vi "Read Magic.vi"(8 "Error In":errorcluster, 11 "Known Host In":refnum<class "Known Host.lvclass">) -> (0 "Error Out":errorcluster, 2 "Magic":i32, 3 "Known Host Out":refnum<class "Known Host.lvclass">)   [LabVIEW 2021, in "Field_RnD_Services_LIBSSH2_Toolkit.lvlib" / "Known Host.lvclass"]
doc: "Gets the \"magic\" number that is part of the libssh2 shared library implementation of a Known Host struct."
uses:
  Known Host.lvclass
  Known Host.lvclass/Known Host.ctl
  Field_RnD_Services_LIBSSH2_Toolkit.lvlib
  SSH/SSH.lvclass
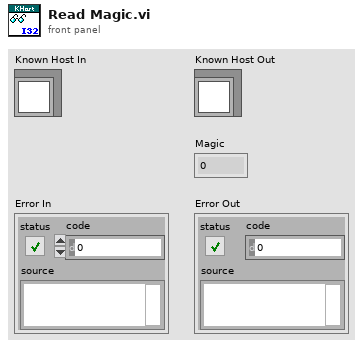
[diagram p1: front panel]
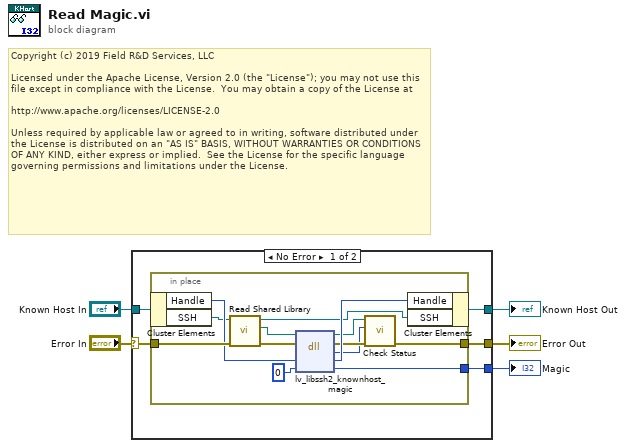
[diagram p0: block diagram]
diagram:
  # "Copyright (c) 2019 Field R&D Services, LLC\n\nLicensed under the Apache License, Version 2.0 (the \"License\"); you may not use this file except in compliance with the License.  You may obtain a copy of the License at\n\nhttp://www.apache.org/licenses/LICENSE-2.0\n\nUnless required by applicable law or agreed to in writing, software distributed under the License is distributed on an \"AS IS\" BASIS, WITHOUT WARRANTIES OR CONDITIONS OF ANY KIND, either express or implied.  See the License for the specific language governing permissions and limitations under the License."
  n1 = case shown="No Error" "Error In" {
    selector: "Error In" -> [w10 w25]
    tunnel: [w9 w25] -> w4
    tunnel: "Known Host In" -> [w8 w24]
    tunnel: [w7 w24] -> w2
    tunnel: [w6 _] -> w1
    frame No Error {
      n2 = in-place {
        in-place-border: w10 -> [w23]
        in-place-border: [w18] -> w9
        in-place-border: [w15] -> w6
        n3 = in-place-cluster #1(w8) -> ("Handle"=w22:u64, "SSH"=w13:refnum<class "SSH.lvclass">)
        n4 = call "Read Shared Library.vi"("Error In"=w23, "SSH In"=w13) -> ("Error Out"=w14:errorcluster, "libssh2lv Shared Library"=w12:path, "SSH Out"=w11:refnum<class "SSH.lvclass">)  [unwired: 7 in]
        n5 = dll-call lib="lv-libssh2.*" fn="lv_libssh2_knownhost_magic"(path in=w12, error in=w14, "handle"=w22, "magic"=0) -> (path out=w17:path, error out=w19:errorcluster, "status"=w16:i32, "handle"=w21:u64, "magic"=w15:i32)  [unwired: 1 in]
        n6 = call "Check Status.vi"("Error In"=w19, "Status"=w16, "libssh2lv Shared Library In"=w17) -> ("Error Out"=w18:errorcluster)  [unwired: 7 in, 1 out]
        n7 = in-place-cluster #1("Handle"=w21, "SSH"=w11) -> (w7:refnum<class "Known Host.lvclass">)
      }
    }
    frame Error {
    }
  }
  "Error Out" <- w4
  "Known Host Out" <- w2
  "Magic" <- w1
